vi "Exercise 3 Solution.vi"() -> ()   [LabVIEW 2019]
panel:
  in  "Number of Samples":i32=10
  out "Sum":dbl format="%#_5g"
  in  "Limit":dbl=9.0
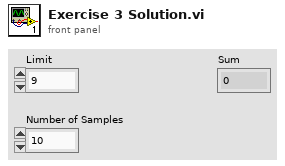
[diagram p1: front panel]
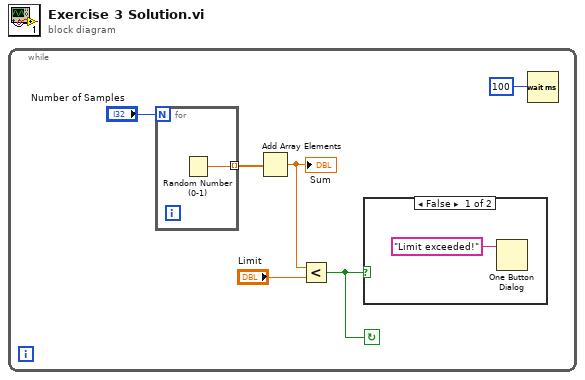
[diagram p0: block diagram]
diagram:
  n1 = while {
    stop <- w4 continue-if-true
    n2 = for {
      N: "Number of Samples" -> [_]
      tunnel: [w8] -> w2 mode=indexing
      n3 = Random Number (0-1)() -> (number: 0 to 1=w8:dbl)
    }
    n4 = Add Array Elements(numeric array=w2) -> (sum=w1:dbl)
    "Sum" <- w1
    n5 = Less?(x=w1, y="Limit") -> (x < y?=w4:bool)
    n6 = case shown="False" w4 {
      frame False {
        n7 = One Button Dialog(message="Limit exceeded!") -> ()  [unwired: 1 in, 1 out]
      }
      frame True {
      }
    }
    n8 = Wait (ms)(milliseconds to wait=u32 100) -> ()  [unwired: 1 out]
  }
